vi "KCP.vi"(0 "System no.":i32=1 min=1 max=4 step=1, 2 "Source CS":string, 3 "Destination CS":string, 5 "error in":errorcluster) -> (19 "error out":errorcluster)   [LabVIEW 2020]
doc: "Copies a coordinate system (e. g. in order to create a backup copy), and queries ERR?. Controller error is TRUE if selected system reports error code not equal to 0.\n\nC-887, F-206, M-8X0: Only for GCS syntax version = GCS 2.0 or higher (Check with CSV?.vi. If CSV?.vi is not supported, syntax version is GCS 1.0)."
panel:
  # "Copies a coordinate system (e. g. in order to create a backup copy),  and \nqueries for ERR?."
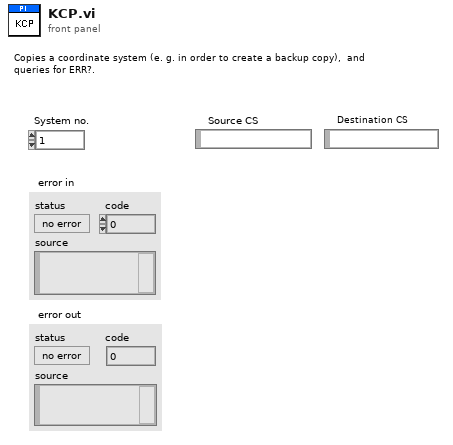
[diagram p1: front panel]
types:
  T1 = enum16{"Disable error check", "Force error check", "Use global settings"}
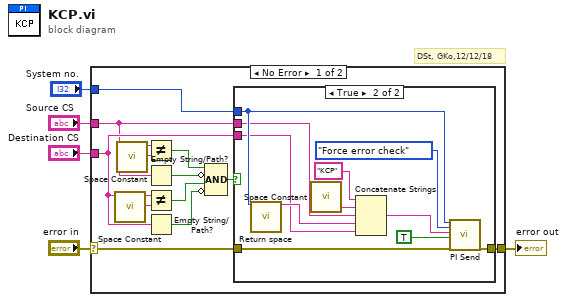
[diagram p0: block diagram]
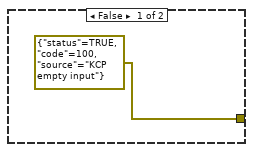
[diagram p2: hidden frame]
diagram:
  # "DSt, GKo,12/12/18"
  n1 = case shown="No Error" "error in" {
    selector: "error in" -> [w12 w30]
    tunnel: "Source CS" -> [w8 _]
    tunnel: [w11 w30] -> w5
    tunnel: "Destination CS" -> [w10 _]
    tunnel: "System no." -> [w17 _]
    frame No Error {
      n2 = call <vilib>:"Space Constant.vi"() -> ("String"=w15:string)
      n3 = call <vilib>:"Space Constant.vi"() -> ("String"=w16:string)
      n4 = Not Equal?(x=w8, y=w16) -> (x != y?=w14:bool)
      n5 = Empty String/Path?(string/path=w8) -> (empty?=w7:bool)
      n6 = Not Equal?(x=w10, y=w15) -> (x != y?=w13:bool)
      n7 = Empty String/Path?(string/path=w10) -> (empty?=w9:bool)
      n8 = Compound Arithmetic op=AND(w14, invert w7, w13, invert w9) -> (w6:bool)
      n9 = case shown="True" w6 {
        tunnel: w17 -> [_ w29]
        tunnel: w12 -> [_ w28]
        tunnel: [errorcluster {"status"=TRUE, "code"=100, "source"="KCP empty input"} ("error out") w27] -> w11
        tunnel: w10 -> [_ w19]
        tunnel: w8 -> [_ w21]
        frame False {
        }
        frame True {
          n10 = call "Return space.vi"("System no."=w29) -> ("String out"=w20:string)  [unwired: 1 in, 17 out]
          n11 = call <vilib>:"Space Constant.vi"() -> ("String"=w22:string)
          n12 = Concatenate Strings("KCP", w22, w21, w20, w19) -> (w24:string)
          n13 = call "PI Send.vi"("System no."=w29, "Error check settings"=T1."Force error check", "String to send"=w24, "Attach termination char.?"=TRUE ("Attach Linefeed?"), "error in"=w28) -> ("error out"=w27:errorcluster)  [unwired: 1 in, 13 out]
        }
      }
    }
    frame Error {
    }
  }
  "error out" <- w5
